vi "ScriptEventMenuActivation.vi"(8 "error in (no error)":errorcluster, 9 "rowIndex":i32, 10 "MenuRef":refnum<k9>, 11 "ScriptEditorV2 in":refnum<class "ScriptEditorV2.lvclass">) -> (0 "error out":errorcluster, 3 "ScriptEditorV2 out":refnum<class "ScriptEditorV2.lvclass">)   [LabVIEW 2009, in "Views.lvlib" / "ScriptEditor.lvlib" / "ScriptEditorV2.lvclass"]
uses:
  ScriptEditorV2.lvclass
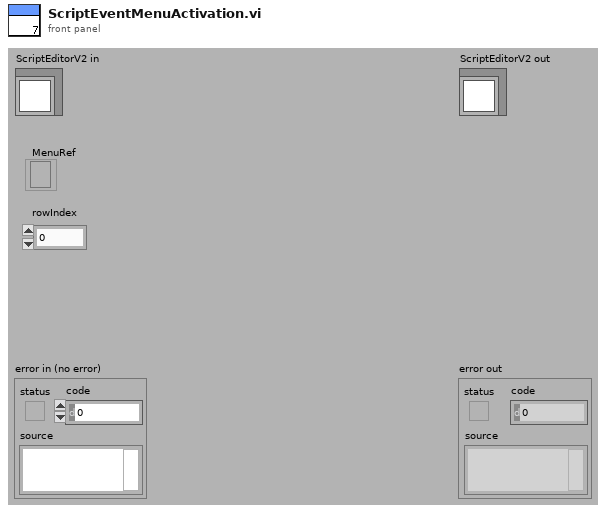
[diagram p1: front panel]
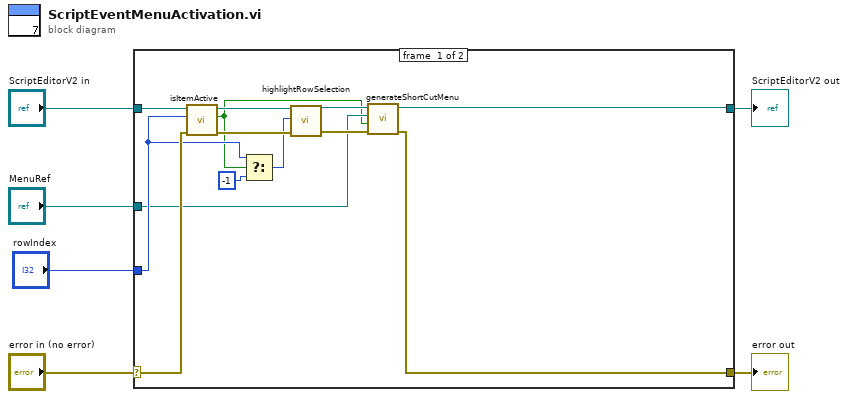
[diagram p0: block diagram]
diagram:
  n1 = case shown="No Error" "error in (no error)" {
    selector: "error in (no error)" -> [w18 w21]
    tunnel: [w7 w21] -> w5
    tunnel: [w11 w20] -> w3
    tunnel: "ScriptEditorV2 in" -> [w19 w20]
    tunnel: "MenuRef" -> [w9 _]
    tunnel: "rowIndex" -> [w15 _]
    frame #0 {
      n2 = call "isItemActive.vi"("error in (no error)"=w18, "rowIndex"=w15, "ScriptEditorV2 in"=w19) -> ("error out"=w16:errorcluster, "active"=w8:bool, "ScriptEditorV2 out"=w17:refnum<class "ScriptEditorV2.lvclass">)  [unwired: 6 in]
      n3 = Select(t=w15, s=w8, f=-1) -> (s? t:f=w14:i32)
      n4 = call "highlightRowSelection.vi"("error in (no error)"=w16, "rowIndex"=w14, "ScriptEditorV2 in"=w17) -> ("error out"=w10:errorcluster, "ScriptEditorV2 out"=w12:refnum<class "ScriptEditorV2.lvclass">)  [unwired: 7 in]
      n5 = call "generateShortCutMenu.vi"("error in (no error)"=w10, "activeRow?"=w8, "MenuRef"=w9, "ScriptEditorV2 in"=w12) -> ("error out"=w7:errorcluster, "ScriptEditorV2 out"=w11:refnum<class "ScriptEditorV2.lvclass">)  [unwired: 6 in]
    }
    frame #1 {
    }
  }
  "error out" <- w5
  "ScriptEditorV2 out" <- w3
